vi "Wash Process.vi"(11 "Wash Options":T2) -> (3 "Array":T1[](array[typedef]))   [LabVIEW 2018]
uses:
  Controls/Wash Options.ctl
  Controls/States Enum.ctl
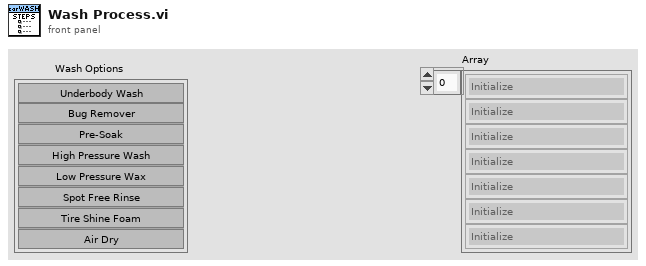
[diagram p1: front panel]
types:
  T1 = typedef "States Enum.ctl" = enum16{"Initialize", "WaitEvent", "Stop", "UnderBodyWash", "BugRemover", "PreSoak", "HighPressureWash", "LowPressureWash", "SpotFreeRinse", "TireShineFoam", "AirDry"}
  T2 = typedef "Wash Options.ctl" = cluster{"Underbody Wash":bool, "Bug Remover":bool, "Pre-Soak":bool, "High Pressure Wash":bool, "Low Pressure Wax":bool, "Spot Free Rinse":bool, "Tire Shine Foam":bool, "Air Dry":bool}
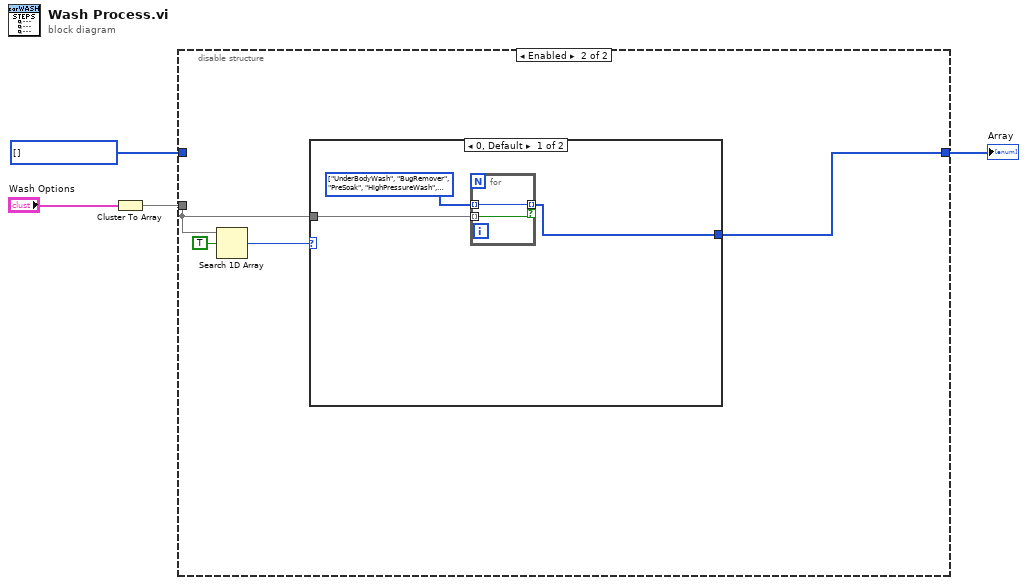
[diagram p0: block diagram]
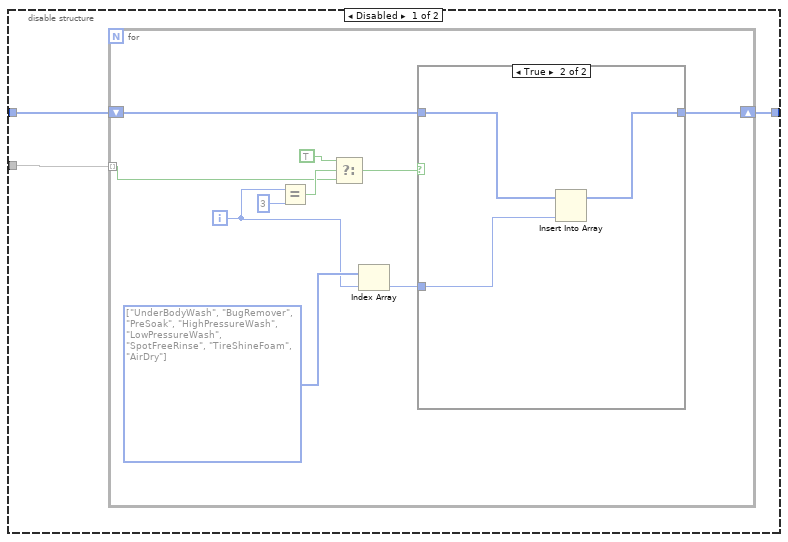
[diagram p2: hidden frame]
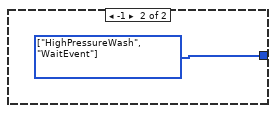
[diagram p4: hidden frame]
diagram:
  w2 = T1[] [] items=["Initialize", "WaitEvent", "Stop", "UnderBodyWash", "BugRemover", "PreSoak", "HighPressureWash", "LowPressureWash", "SpotFreeRinse", "TireShineFoam", "AirDry"] ("Array")
  n1 = Cluster To Array(cluster="Wash Options") -> (array=w3:bool[])
  n2 = disable-structure shown="Enabled" {
    disable-tunnel: w3 -> [w7 w22]
    disable-tunnel: w2 -> [w6 _]
    disable-tunnel: [w5 w23] -> w1
    frame Disabled {
      n3 = for {
        tunnel: w7 -> [w8] mode=indexing
        shift-right: [w15] -> w5
        shift-left: w6 -> [w14]
        i -> [w13]
        w17 = T1[] [enum."UnderBodyWash", enum."BugRemover", enum."PreSoak", enum."HighPressureWash", enum."LowPressureWash", enum."SpotFreeRinse", enum."TireShineFoam", enum."AirDry"] items=["Initialize", "WaitEvent", "Stop", "UnderBodyWash", "BugRemover", "PreSoak", "HighPressureWash", "LowPressureWash", "SpotFreeRinse", "TireShineFoam", "AirDry"] ("Array")
        n4 = Equal?(x=w13, y=3) -> (x = y?=w11:bool)
        n5 = Select(t=TRUE, s=w11, f=w8) -> (s? t:f=w9:bool)
        n6 = Index Array(array=w17, index=w13) -> (element=w16:T1)
        n7 = case shown="True" w9 {
          tunnel: w16 -> [_ w21]
          tunnel: [w18 w20] -> w15
          tunnel: w14 -> [w18 w19]
          frame False {
          }
          frame True {
            n8 = Insert Into Array(array=w19, new element=w21) -> (w20:T1[])  [unwired: 1 in]
          }
        }
      }
    }
    frame Enabled {
      n9 = Search 1D Array(1D array=w22, element=TRUE) -> (index of element=w24:i32)  [unwired: 1 in]
      n10 = case shown="0, Default" w24 {
        tunnel: [w26 w31] -> w23
        tunnel: w22 -> [w28 _]
        frame 0, Default {
          w27 = T1[] [enum."UnderBodyWash", enum."BugRemover", enum."PreSoak", enum."HighPressureWash", enum."LowPressureWash", enum."SpotFreeRinse", enum."TireShineFoam", enum."AirDry"] items=["Initialize", "WaitEvent", "Stop", "UnderBodyWash", "BugRemover", "PreSoak", "HighPressureWash", "LowPressureWash", "SpotFreeRinse", "TireShineFoam", "AirDry"] ("Array")
          n11 = for {
            tunnel: w28 -> [w29] mode=indexing
            tunnel: [w30] -> w26 mode=indexing if=w29
            tunnel: w27 -> [w30] mode=indexing
          }
        }
        frame -1 {
          w31 = T1[] [enum."HighPressureWash", enum."WaitEvent"] items=["Initialize", "WaitEvent", "Stop", "UnderBodyWash", "BugRemover", "PreSoak", "HighPressureWash", "LowPressureWash", "SpotFreeRinse", "TireShineFoam", "AirDry"] ("Array")
        }
      }
    }
  }
  "Array" <- w1
